vi "Dashboard Main Old.vi"() -> ()   [LabVIEW 2015]
uses:
  <vilib>/Utility/miscctls.llb/LVRowAndColumnTypeDef.ctl
  <vilib>/event_ctls.llb/eventvkey.ctl
  <vilib>/Rock Robotics/WPI/Dashboard/WPI_DashboardLogging Global.vi
  <vilib>/Rock Robotics/Network Tables/NT Write Boolean.vi
  <vilib>/Utility/config.llb/Write Key (String).vi
  <vilib>/Utility/config.llb/Write Key (I32).vi
  <vilib>/Utility/config.llb/NI_LVConfig.lvlib
panel:
  in  "TCP":refnum<k5>
  in  "Rec Mode":enum32{"Stop", "Record", "Playback"}(radio)
  in  "Vision":u16(ring)=2 items=["Camera Off", "USB Camera SW", "USB Camera HW", "IP Camera"]
  out "Camera IP":string
  out "Image Message":string="Timeout in Camera Communications"
  in  "Dashboard Tab":T1(tab)
  out "NT Connection":bool
  in  "Camera Settings":T2={"Frame Rate"=30, "Compression"=30, "Size"=1} {"Frame Rate" scale=1.0..30.0; "Size" items=["640x480", "320x240", "160x120"]}
  out "Gyro":dbl(knob) scale=0.0..360.0
  out "Mode":T3(ring)=enum."Auto Disabled"
  in  "DB Camera Config":bool
  out "fps":dbl format="%#.1g"
  out "Mbps":dbl format="%#.1g"
  out "Mbps LED":bool
  in  "DB/String 9":string
  in  "DB/String 8":string
  in  "DB/String 7":string
  in  "DB/String 6":string
  in  "DB/String 5":string
  in  "DB/String 4":string
  in  "DB/String 3":string
  in  "DB/String 2":string
  in  "DB/String 1":string
  in  "DB/String 0":string
  in  "DB/Slider 0":dbl(slide) scale=0.0..5.0
  in  "DB/Slider 1":dbl(slide) scale=0.0..5.0
  in  "DB/Slider 2":dbl(slide) scale=0.0..5.0
  in  "DB/Slider 3":dbl(slide) scale=0.0..5.0
  out "DB/LED 3":bool
  out "DB/LED 2":bool
  out "DB/LED 1":bool
  out "DB/LED 0":bool
  in  "DB/Button 3":bool
  in  "DB/Button 2":bool
  in  "DB/Button 1":bool
  in  "DB/Button 0":bool caption="New Name"
  in  "Auto Mode":u16(ring) items=["Do Nothing", "Drive to OW", "Drive through OW", "Shoot"]
  in  "Select Auto":string(combo)="Do Nothing"
  in  "Starting Position":u16(ring) items=["1", "2", "3", "4", "5", "Spy"]
  in  "Defense to Cross":u16(ring) items=["Low Bar", "Moat", "Ramparts", "Rock Wall", "Rough Terrain", "Cheval", "Portculis"]
  in  "Shooter Towards Defense":bool
  in  "Test Slider":dbl(slide) scale=0.0..100.0 scale format="%#_3g"
  in  "On/Off":bool caption="Solenoid"
  in  "Test Name":u16(ring) items=["Select the test to run..."]
  in  "Test Tree":string(tree)
  in  "Motor":cluster{"Value":dbl, "Enable":bool} {"Value" scale=-1.0..1.0 scale format="%#_3g"}
  out "Progress":T4 {"Test Progress" scale=0.0..100.0}
  in  "Rev/Fwd":cluster{"Forward":bool, "Reverse":bool}
  in  "Test Ring":u16(ring) items=["Monochrome", "Color"]
  out "Cmd Status":string
  in  "Execute Command":bool
  in  "Command Params":string[][](table)
  in  "Command Selection":i32(listbox)
  in  "CheckList":i32(listbox)
  out "Tree":string(tree)
  out "Camera Image":T5(plugin-control)
  out "Background":bool
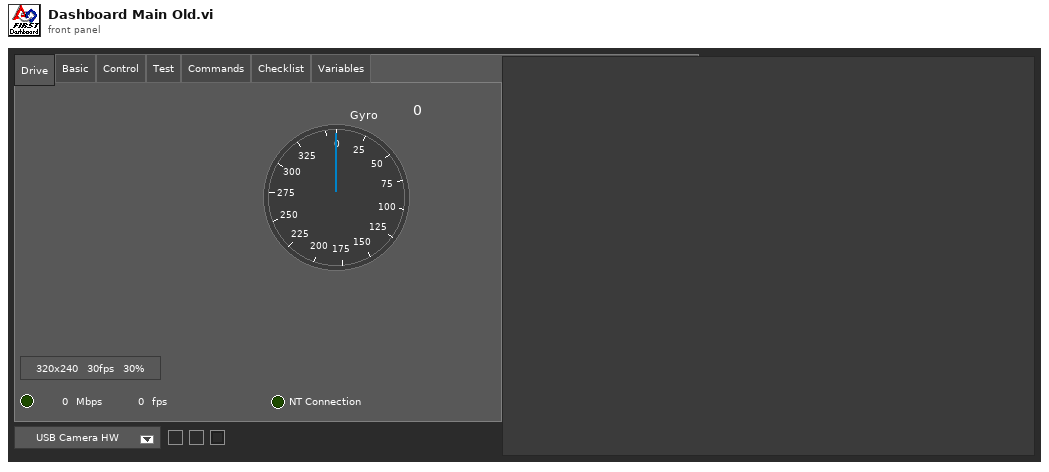
[diagram p1: front panel]
types:
  T1 = enum32{"Drive", "Basic", "Control", "Test", "Commands", "Checklist", "Variables"}
  T2 = cluster{"Frame Rate":i32, "Compression":i32, "Size":u16}
  T3 = enum8{"Tele-Op Disabled", "Tele-Op Enabled", "Auto Disabled", "Auto Enabled", "Test Disabled", "Test Enabled", "Disconnected", "No Code", "E-Stop"}
  T4 = cluster{"Test Progress":u8, "Test Progress Text":string}
  T5 = typedef "IMAQ Image.ctl" = refnum<image>
  T6 = cluster{"IDs":cluster{"RPC field ID":u16, "Unique ID":u16}, "String":string}
  T7 = enum32{"Drive", "Basic", "Custom", "Test", "Checklist", "Variables"}
  T8 = typedef "Image Type" = u32
  T9 = cluster{"Camera Image":refnum<vi>, "Dashboard Tab":refnum<vi>, "Background":refnum<vi>, "Vision":refnum<vi>, "Rec Mode":refnum<vi>, "Test Slider":refnum<vi>, "On/Off ":refnum<vi>, "Test Ring":refnum<vi>, "Rev/Fwd":refnum<vi>, "Test Name":refnum<vi>, "Motor":refnum<vi>, "Progress":refnum<vi>, "CheckList":refnum<vi>, "Tree":refnum<vi>, "Test Tree":refnum<vi>, "Command Params":refnum<vi>, "Command Selection":refnum<vi>, "Execute Command":refnum<vi>, "Cmd Status":refnum<vi>}
  T10 = cluster{"Error Strings":string, "Disable Counts":cluster{u16, u16}, "Rail Faults":cluster{u16, u16, u16}, "Robot IP":string, "DB Mode":u8, "Event Info":cluster{"Name":string, "Type":u8, "Number":u16, "Replay":u8}, "Camera Addr":string}
  T11 = cluster{"Storage":cluster{"Disk Free":u64, "RAM Block":u32, "RAM free":u32}, "CPU Utilization":cluster{"CPU % ISR":sgl, "CPU % Time Crit":sgl, "CPU % Timed Str":sgl, "CPU % High":sgl, "CPU % Above":sgl, "CPU % Normal":sgl, "CPU % Low":sgl}, "CAN":cluster{"% Bus Utilization":sgl, "Bus Off Cnt":u32, "TX_FIFO Full Cnt":u32, "Receive Error Cnt":u8, "Transmit Error Cnt":u8}, "HID":cluster{"HID Outputs":u32, "Rumble Low":u16, "Rumble High":u16}[]}
  T12 = cluster{"Status bits":cluster{"Test Mode":bool, "Autonomous":bool, "Enabled":bool, "Code Start":bool, "Brownout":bool, "Reserved 2":bool, "Reserved 3":bool, "E-Stop":bool}, "Code Trace":cluster{"Disabled":bool, "TeleOp":bool, "Auto":bool, "Test":bool}, "Controller Type":enum16{"unknown", "cRIO", "roboRio"}, "Code?":enum16{"unknown", "noCode", "code"}, "Battery V":dbl}
  T13 = cluster{"Control Bits":cluster{"TestMode":bool, "Autonomous":bool, "Enabled":bool, "FMS Present":bool, bool, bool, bool, "E-Stop":bool}, "Team Station ":u8, "Countdown":sgl, "Joystick Values":cluster{"Axes":dbl[], "Buttons":bool[], "POVs":i16[]}[]}
  T14 = typedef "NI_LVConfig.lvlib/Config Data RefNum.ctl" = refnum<k1>
  T15 = cluster{"Operation":enum16{"Update", "Clear"}, "Color Box":u32}[]
  T16 = typedef "eventvkey.ctl" = enum16{"ASCII", "Enter", "Return", "Shift", "Ctrl", "Alt", "Cmd", "Opt", "Caps", "NumLock", "Clear", "Break", "Up", "Down", "Left", "Right", "Insert", "Delete", "Home", "End", "PageUp", "PageDown", "Escape", "Help", "Pause", "ScrollLock", "F1", "F2", "F3", "F4", "F5", "F6", "F7", "F8", "F9", "F10", "F11", "F12", "F13", "F14", "F15", "F16", "F17", "F18", "F19", "F20", "F21", "F22", "F23", "F24", "Play", "VolumeUp", "VolumeDown", "Mute", "Two Byte Char"}
  T17 = cluster{"Image Size":bool, "Image Type":bool, "Pixel Value":bool, "ROI Information":bool, "Zoom Factor":bool}
  T18 = enum8{"Enabled", "Disabled", "Disabled and Grayed Out"}
  T19 = cluster{"Operation":enum16{"Update", "Clear"}, "Color Box":u32}
  T20 = typedef "LVRowAndColumnTypeDef.ctl" = cluster{"Row":i32, "Column":i32}
  T21 = cluster{"Shift":bool, "Ctrl":bool, "Alt":bool, "Cmd":bool, "Opt":bool}
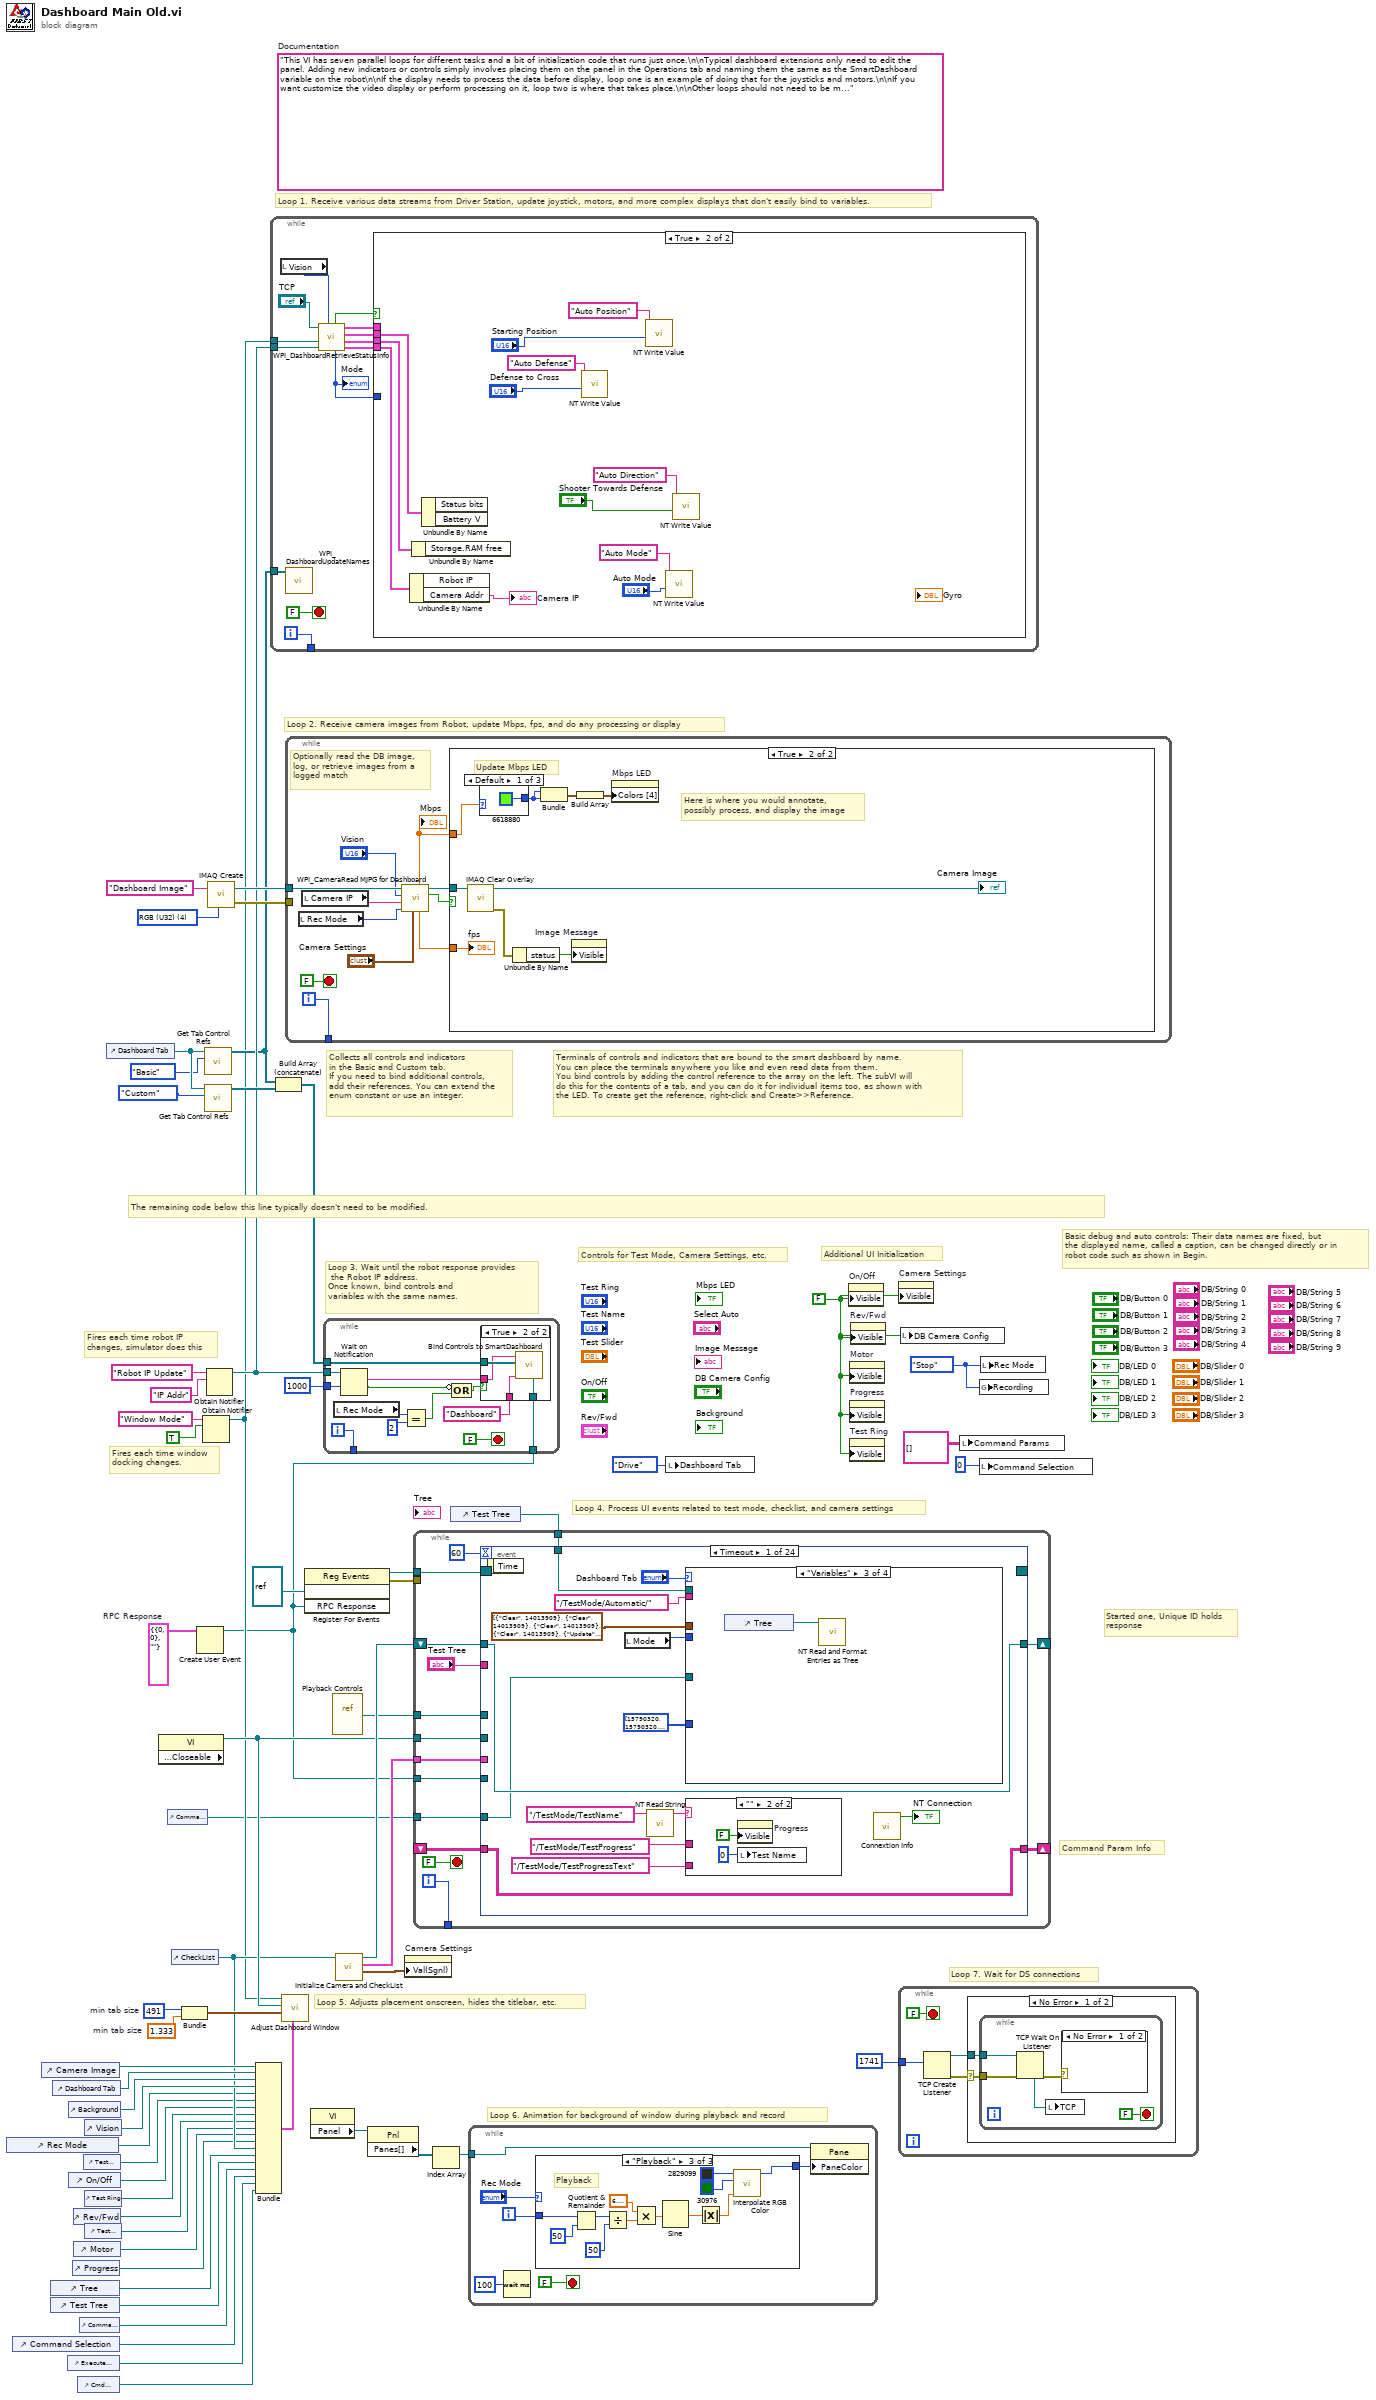
[diagram p0: block diagram]
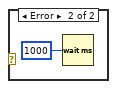
[diagram p2: hidden frame]
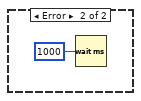
[diagram p3: hidden frame]
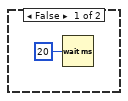
[diagram p4: hidden frame]
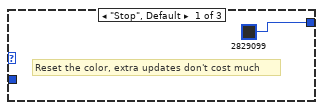
[diagram p5: hidden frame]
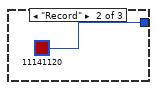
[diagram p6: hidden frame]
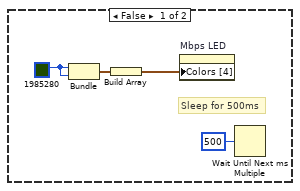
[diagram p8: hidden frame]
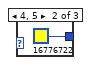
[diagram p9: hidden frame]
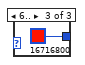
[diagram p10: hidden frame]
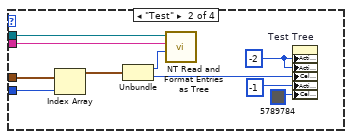
[diagram p12: hidden frame]
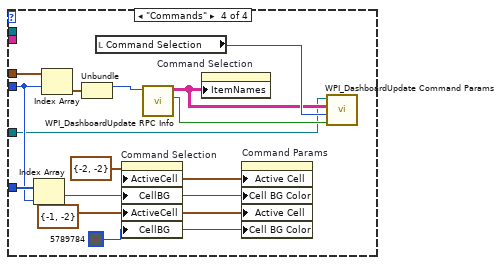
[diagram p13: hidden frame]
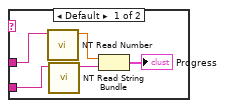
[diagram p14: hidden frame]
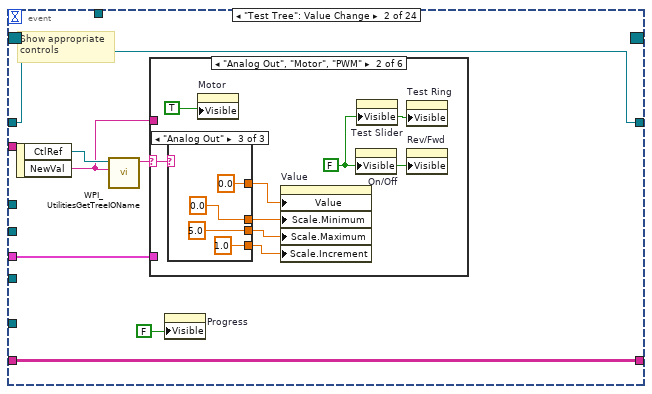
[diagram p15: hidden frame]
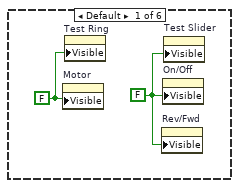
[diagram p16: hidden frame]
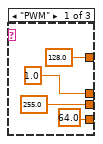
[diagram p17: hidden frame]
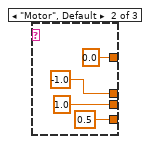
[diagram p18: hidden frame]
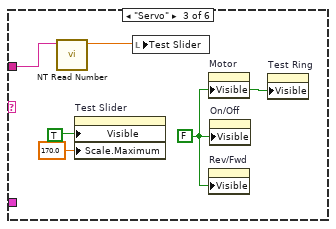
[diagram p19: hidden frame]
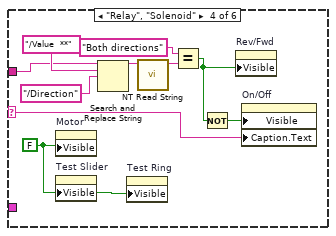
[diagram p20: hidden frame]
diagram:
  w8 = T6 {"IDs"={"RPC field ID"=0, "Unique ID"=0}, "String"=""}  # RPC Response
  w33 = 491  # min tab size
  w32 = 1.333  # min tab size
  w41 = enum32{"Stop", "Record", "Playback"}."Stop" ("Rec Mode")
  w15 = FALSE ("Visible")
  (unwired) "This VI has seven parallel loops for different tasks and a bit of initialization code that runs just once.\n\nTypical dashboard extensions only need to edit the panel. Adding new indicators or controls simply involves placing them on the panel in the Operations tab and naming them the same as the SmartDashboard variable on the robot\n\nIf the display needs to process the data before display, loop one is an example of doing that for the joysticks and motors.\n\nIf you want customize the video display or perform processing on it, loop two is where that takes place.\n\nOther loops should not need to be modified. They are pretty standard, and document the task they perform."  # Documentation
  w61 = T8 4 items=["Grayscale (U8)", "Grayscale (I16)", "Grayscale (SGL)", "Complex (CSG)", "RGB (U32)", "HSL (U32)", "RGB (U64)"] ("Image Type")
  # "Command Param Info"
  # "Started one, Unique ID holds\nresponse"
  # "Loop 7. Wait for DS connections"
  # "Basic debug and auto controls: Their data names are fixed, but\nthe displayed name, called a caption, can be changed directly or in\nrobot code such as shown in Begin."
  # "Controls for Test Mode, Camera Settings, etc."
  # "Additional UI Initialization"
  # "Loop 6. Animation for background of window during playback and record"
  # "Fires each time robot IP\nchanges, simulator does this"
  # "Fires each time window\ndocking changes."
  # "Collects all controls and indicators\nin the Basic and Custom tab.\nIf you need to bind additional controls,\nadd their references. You can extend the\nenum constant or use an integer."
  # "The remaining code below this line typically doesn't need to be modified."
  # "Loop 4. Process UI events related to test mode, checklist, and camera settings"
  # "Terminals of controls and indicators that are bound to the smart dashboard by name.\nYou can place the terminals anywhere you like and even read data from them.\nYou bind controls by adding the control reference to the array on the left. The subVI will\ndo this for the contents of a tab, and you can do it for individual items too, as shown with\nthe LED. To create get the reference, right-click and Create>>Reference."
  # "Loop 3. Wait until the robot response provides\n the Robot IP address.\nOnce known, bind controls and\nvariables with the same names."
  # "Loop 5. Adjusts placement onscreen, hides the titlebar, etc."
  # "Loop 1. Receive various data streams from Driver Station, update joystick, motors, and more complex displays that don't easily bind to variables."
  # "Loop 2. Receive camera images from Robot, update Mbps, fps, and do any processing or display"
  n1 = control-ref of="Rec Mode"() -> (w21:refnum<vi>)
  n2 = control-ref of="Command Selection"() -> (w7:refnum<vi>)
  n3 = control-ref of="Camera Image"() -> (w36:refnum<vi>)
  n4 = control-ref of="Tree"() -> (w25:refnum<vi>)
  n5 = control-ref of="Test Tree"() -> (w24:refnum<vi>)
  n6 = control-ref of="Dashboard Tab"() -> (w35:refnum<vi>)
  n7 = control-ref of="Execute Command"() -> (w9:refnum<vi>)
  n8 = control-ref of="Background"() -> (w30:refnum<vi>)
  n9 = control-ref of="On/Off"() -> (w19:refnum<vi>)
  n10 = control-ref of="Progress"() -> (w16:refnum<vi>)
  n11 = control-ref of="Rev/Fwd"() -> (w17:refnum<vi>)
  n12 = control-ref of="Motor"() -> (w22:refnum<vi>)
  n13 = control-ref of="Cmd Status"() -> (w3:refnum<vi>)
  n14 = control-ref of="Command Params"() -> (w10:refnum<vi>)
  n15 = control-ref of="Test Slider"() -> (w20:refnum<vi>)
  n16 = control-ref of="Vision"() -> (w34:refnum<vi>)
  n17 = control-ref of="Test Ring"() -> (w18:refnum<vi>)
  n18 = control-ref of="Test Name"() -> (w23:refnum<vi>)
  n19 = control-ref of="Dashboard Tab"() -> (w39:refnum<vi>)
  n20 = property class="VI" props=["Front Panel.Closeable"]() -> (reference out=w40:refnum<vi>)  [unwired: 2 in, 2 out]
  n21 = control-ref of="Command Params"() -> (w2:refnum<vi>)
  n22 = control-ref of="CheckList"() -> (w26:refnum<vi>)
  n23 = Bundle("min tab size"=w33, "min tab size"=w32) -> (w31:cluster{"min tab size":i32, "min tab size":dbl})  [unwired: 1 in]
  n24 = Create User Event(user event datatype=w8) -> (user event=w4:refnum<user-event>)  [unwired: 1 in, 1 out]
  n25 = Obtain Notifier(name (unnamed)="Window Mode", notification data type=TRUE) -> (notifier out=w12:refnum<notifier>)  [unwired: 2 in, 2 out]
  n26 = call <vilib>:"Get Tab Control Refs.vi"("Page Index"=T7."Basic" ("Dashboard Tab"), "TabControl in"=w39) -> ("ControlsOnPage"=w13:refnum<vi>[])  [unwired: 9 in]
  n27 = call <vilib>:"Get Tab Control Refs.vi"("Page Index"=T7."Custom" ("Dashboard Tab"), "TabControl in"=w39) -> ("ControlsOnPage"=w38:refnum<vi>[])  [unwired: 9 in]
  n28 = Obtain Notifier(name (unnamed)="Robot IP Update", notification data type="IP Addr" ("name (unnamed)")) -> (notifier out=w14:refnum<notifier>)  [unwired: 2 in, 2 out]
  n29 = call "IMAQ Create"("Image Name"="Dashboard Image", "Image Type"=w61) -> ("New Image"=w59:T5, "error out"=w58:errorcluster)  [unwired: 2 in, 1 out]
  n30 = Bundle("Camera Image"=w36, "Dashboard Tab"=w35, "Background"=w30, "Vision"=w34, "Rec Mode"=w21, "Test Slider"=w20, "On/Off"=w19, "Test Ring"=w18, "Rev/Fwd"=w17, "Test Name"=w23, "Motor"=w22, "Progress"=w16, "CheckList"=w26, "Tree"=w25, "Test Tree"=w24, "Command Params"=w10, "Command Selection"=w7, "Execute Command"=w9, "Cmd Status"=w3) -> (w27:T9)  [unwired: 1 in]
  n31 = while {
    tunnel: [w73] -> _
    tunnel: w14 -> [w67]
    tunnel: w13 -> [w66]
    tunnel: w12 -> [w62]
    i -> [w73]
    stop <- FALSE stop-if-true
    n32 = local read "Vision"() -> (w64:u16)
    n33 = call <vilib>:"WPI_DashboardUpdateNames.vi"("Controls on Tab"=w66) -> ()  [unwired: 11 in]
    n34 = call <vilib>:"WPI_DashboardRetrieveStatusInfo.vi"("Vision"=w64, "Binding Refnum"=w67, "Window Mode Notifier"=w62, "TCP Cnx"="TCP") -> ("Power and Errors"=w68:T10, "Robot Metrics"=w71:T11, "Status Info"=w72:T12, "Control Info"=w69:T13, "Robot Mode"=w65:T3, "Process?"=w70:bool)  [unwired: 2 in]
    "Mode" <- w65
    n35 = case shown="True" w70 {
      tunnel: w72 -> [_ w87]
      tunnel: w71 -> [_ w86]
      tunnel: w69 -> [_ _]
      tunnel: w68 -> [_ w85]
      tunnel: w65 -> [_ _]
      frame False {
        n36 = Wait (ms)(milliseconds to wait=u32 20) -> ()  [unwired: 1 out]
      }
      frame True {
        n37 = Unbundle By Name(w85) -> ("Camera Addr"=→"Camera IP":string)  [unwired: 1 out]
        n38 = Unbundle By Name(w86) -> ()  [unwired: 1 out]
        n39 = Unbundle By Name(w87) -> ()  [unwired: 2 out]
        n40 = call-poly <vilib>:"NT Write Value.vi"("Numeric"="Defense to Cross", "Name"="Auto Defense") -> ()  [unwired: 9 in, 1 out]
        n41 = call-poly <vilib>:"NT Write Value.vi"("Numeric"="Starting Position", "Name"="Auto Position") -> ()  [unwired: 9 in, 1 out]
        n42 = call-poly <vilib>:"NT Write Value.vi"("Numeric"="Auto Mode", "Name"="Auto Mode") -> ()  [unwired: 9 in, 1 out]
        n43 = call-poly <vilib>:"NT Write Value.vi"("Boolean"="Shooter Towards Defense", "Name"="Auto Direction") -> ()  [unwired: 9 in, 1 out]
      }
    }
  }
  n44 = Build Array (concatenate)(w13, w38) -> (w37:refnum<vi>[])
  n45 = call "Adjust Dashboard Window.vi"("Sizing Refnums"=w27, "Size Constraints"=w31, "VI"=w40, "WIn Mode"=w12) -> ()  [unwired: 8 in]
  n46 = while {
    tunnel: w59 -> [w96]
    tunnel: w58 -> [_]
    tunnel: [w97] -> _
    i -> [w97]
    stop <- FALSE stop-if-true
    # "Optionally read the DB image,\nlog, or retrieve images from a\nlogged match"
    n47 = local read "Rec Mode"() -> (w91:enum32{"Stop", "Record", "Playback"})
    n48 = local read "Camera IP"() -> (w89:string)
    n49 = call <vilib>:"WPI_CameraRead MJPG for Dashboard.vi"("Camera Settings"="Camera Settings", "Rec Mode"=w91, "Camera IP"=w89, "Camera Mode"="Vision", "Refnum in"=w96) -> ("Active"=w94:bool, "Refnum out"=w95:T5, "FPS"=w93:dbl, "Bandwidth (Mbps)"=w88:dbl)  [unwired: 3 in]
    "Mbps" <- w88
    n50 = case shown="True" w94 {
      tunnel: w95 -> [_ w106]
      tunnel: w88 -> [_ w105]
      tunnel: w93 -> [_ w104]
      frame False {
        w99 = u32 1985280 ("Color Box")
        # "Sleep for 500ms"
        n51 = Bundle("Color Box"=w99, "Color Box"=w99) -> (w101:cluster{"Color Box":u32, "Color Box":u32})  [unwired: 1 out]
        n52 = Build Array(w101) -> (w100:cluster{"Color Box":u32, "Color Box":u32}[])
        n53 = property on="Mbps LED" class="Bool (strict)"("Colors [4]"=w100) -> ()  [unwired: 2 in, 2 out]
        n54 = Wait Until Next ms Multiple(millisecond multiple=u32 500) -> ()  [unwired: 1 out]
      }
      frame True {
        # "Here is where you would annotate,\npossibly process, and display the image"
        # "Update Mbps LED"
        n55 = call "IMAQ Clear Overlay"("Image"=w106) -> ("error out"=w110:errorcluster, "Image Out"=→"Camera Image":T5)  [unwired: 2 in, 7 out]
        n56 = case shown="Default" w105 {
          tunnel: [u32 6618880 ("Color Box") u32 16776722 ("Color Box") u32 16716800 ("Color Box")] -> w107
          frame Default {
          }
          frame 4, 5 {
          }
          frame 6.. {
          }
        }
        n57 = Unbundle By Name(w110) -> ("status"=w111:bool)
        n58 = Bundle("Color Box"=w107, "Color Box"=w107) -> (w109:cluster{"Color Box":u32, "Color Box":u32})  [unwired: 1 out]
        n59 = property on="Image Message" class="Str"("Visible"=w111) -> ()  [unwired: 2 in, 2 out]
        n60 = Build Array(w109) -> (w108:cluster{"Color Box":u32, "Color Box":u32}[])
        n61 = property on="Mbps LED" class="Bool (strict)"("Colors [4]"=w108) -> ()  [unwired: 2 in, 2 out]
        "fps" <- w104
      }
    }
  }
  n62 = register-events(refnum<vi> refnum, w4) -> (reference out=w45:refnum<event-registration>, error out=w44:errorcluster)  [unwired: 2 in]
  n63 = property class="VI"() -> ("Panel"=w48:refnum<vi>)  [unwired: 2 in, 2 out]
  n64 = while {
    tunnel: w37 -> [w127]
    tunnel: w14 -> [w125]
    tunnel: [w123] -> _
    tunnel: u32 1000 ("milliseconds to wait") -> [w122]
    tunnel: w4 -> [w115]
    i -> [w123]
    stop <- FALSE stop-if-true
    n65 = local read "Rec Mode"() -> (w118:enum32{"Stop", "Record", "Playback"})
    n66 = Wait on Notification(notifier=w125, timeout in ms (-1)=w122) -> (notification=w124:string, timed out?=w120:bool)  [unwired: 2 in, 2 out]
    n67 = Equal?(x=w118, y=u16 2 ("Rec Mode")) -> (x = y?=w119:bool)
    n68 = Compound Arithmetic op=OR(invert w120, w119) -> (w121:bool)
    n69 = case shown="True" w121 {
      tunnel: w127 -> [_ w131]
      tunnel: w124 -> [_ w130]
      tunnel: "Dashboard" -> [_ w129]
      tunnel: w115 -> [_ w128]
      frame False {
      }
      frame True {
        n70 = call <vilib>:"Bind Controls to SmartDashboard.vi"("RPC ref"=w128, "Client Name"=w129, "Bound Control Refs"=w131, "Server IP Address"=w130) -> ()  [unwired: 8 in]
      }
    }
  }
  n71 = vi-ref "Playback Controls.vi"() -> (w46:refnum<vi>)
  n72 = call "Initialize Camera and CheckList.vi"("ListBox in"=w26) -> ("Cluster"=w52:cluster{"value":i32, "value":i32, "index":i32}, "Array"=w53:cluster{string[]}[], "File Refnum"=w51:T14)  [unwired: 8 in]
  n73 = property class="Pnl"(reference=w48) -> ("Panes[]"=w49:refnum<vi>[])  [unwired: 1 in, 2 out]
  n74 = property on="Camera Settings" class="Clust (strict)"("Val(Sgnl)"=w52) -> ()  [unwired: 2 in, 2 out]
  n75 = Index Array(array=w49) -> (element=w47:refnum<vi>)  [unwired: 1 in]
  n76 = control-ref of="Test Tree"() -> (w50:refnum<vi>)
  n77 = while {
    tunnel: w53 -> [w143]
    shift-right: [w142] -> _
    shift-left: w51 -> [w141]
    tunnel: [w140] -> _
    tunnel: w50 -> [w139]
    tunnel: w46 -> [w138]
    tunnel: w45 -> [w137]
    tunnel: w44 -> [_]
    tunnel: w40 -> [w136]
    tunnel: w4 -> [w135]
    tunnel: w2 -> [w134]
    shift-right: [w133] -> _
    shift-left: _ -> [w132]
    i -> [w140]
    stop <- FALSE stop-if-true
    n78 = event shown="[0] Timeout" {
      selector: w137 -> [_ _ _ _ _ _ _ _ _ _ _ _ _ _ _ _ _ _ _ _ _ _ _ _]
      dyn-events: [_ _ _ _ _ _ _ _ _ _ _ _ _ _ _ _ _ _ w452 _ _ _ _ _] -> _
      timeout: u32 60 ("milliseconds to wait") -> [_ _ _ _ _ _ _ _ _ _ _ _ _ _ _ _ _ _ _ _ _ _ _ _]
      tunnel: w139 -> [w156 _ _ _ _ _ _ _ _ _ _ _ _ _ _ _ _ _ _ _ _ _ _ _]
      tunnel: "Test Tree" -> [_ _ _ _ _ _ _ _ _ _ _ _ _ w415 w424 w427 w432 w441 _ _ _ _ _ _]
      tunnel: w143 -> [_ w194 _ _ _ _ _ _ _ _ _ w377 w408 _ _ _ _ _ _ _ _ _ _ _]
      tunnel: [w153 w193 w297 w303 w313 w317 w323 w335 w343 w349 w362 w376 w401 w414 w422 w426 w431 w440 w454 w470 w472 w480 w491 w496] -> w142
      tunnel: w141 -> [w153 w193 w297 w303 w313 w317 w323 w335 w343 w349 w362 w375 w401 w414 w422 w426 w431 w440 w454 w470 w472 w480 w491 w496]
      tunnel: w138 -> [_ _ _ _ _ _ _ _ _ _ _ _ _ _ _ _ _ _ w455 _ w475 _ _ _]
      tunnel: w136 -> [_ _ _ _ _ _ _ _ _ _ _ _ _ _ _ _ _ _ w450 _ _ _ _ _]
      tunnel: w135 -> [_ _ _ _ _ _ _ _ _ _ _ _ _ _ _ _ _ _ w446 _ _ _ _ _]
      tunnel: w134 -> [w148 _ _ _ _ _ w321 _ _ _ _ _ _ _ _ _ _ _ _ _ _ _ _ _]
      tunnel: [w147 w192 w296 w302 w312 w318 w319 w329 w340 w348 w361 w374 w400 w413 w421 w425 w430 w439 w445 w468 w471 w476 w484 w497] -> w133
      tunnel: w132 -> [w147 w192 w296 w302 w312 w318 w319 _ _ w348 w361 w374 w400 w413 w421 w425 w430 w439 w445 w468 w471 w476 w484 w497]
      event Timeout {
        n79 = event-data() -> ()  [unwired: 1 in, 1 out]
        n80 = local read "Mode"() -> (w150:T3)
        n81 = call <vilib>:"NT Read String.vi"("Name"="/TestMode/TestName") -> ("String"=w159:string)  [unwired: 9 in, 1 out]
        n82 = case shown="\"Variables\"" "Dashboard Tab" {
          tunnel: w156 -> [_ w170 _ _]
          tunnel: "/TestMode/Automatic/" ("Name Pattern") -> [_ w169 _ _]
          tunnel: T15 [{"Operation"=enum."Clear", "Color Box"=14013909}, {"Operation"=enum."Clear", "Color Box"=14013909}, {"Operation"=enum."Clear", "Color Box"=14013909}, {"Operation"=enum."Clear", "Color Box"=14013909}, {"Operation"=enum."Update", "Color Box"=14013909}, {"Operation"=enum."Update", "Color Box"=16777215}, {"Operation"=enum."Clear", "Color Box"=14013909}, {"Operation"=enum."Clear", "Color Box"=14013909}, {"Operation"=enum."Clear", "Color Box"=14013909}] -> [_ w162 _ w179]
          tunnel: w150 -> [_ w161 _ w178]
          tunnel: u32[] [15790320, 15790320, 15790320, 15790320, 16777215, 16777215, 15790320, 15790320, 15790320] -> [_ _ _ w184]
          tunnel: w148 -> [_ _ _ w172]
          frame "Control", Default {
          }
          frame "Test" {
            w168 = -2 ("Active Item:Row Number")
            n83 = Index Array(array=w162, index=w161) -> (element=w163:T19)
            n84 = Unbundle(w163) -> ("Operation"=w164:enum16{"Update", "Clear"}, "Color Box"=w165:u32)
            n85 = call <vilib>:"NT Read and Format Entries as Tree.vi"("Operation"=w164, "Name Pattern"=w169, "Tree Refnum"=w170) -> ()  [unwired: 7 in, 2 out]
            n86 = property on="Test Tree" class="Tree (strict)"("Active Item Row Number"=w168, "ActiveColNum"=w168, "CellBG"=w165, "Active Item Row Number"=-1 ("Active Item:Row Number"), "CellBG"=u32 5789784 ("Color Box")) -> ()  [unwired: 2 in, 2 out]
          }
          frame "Variables" {
            n87 = control-ref of="Tree"() -> (w171:refnum<vi>)
            n88 = call <vilib>:"NT Read and Format Entries as Tree.vi"("Tree Refnum"=w171) -> ()  [unwired: 9 in, 2 out]
          }
          frame "Commands" {
            w180 = u32 5789784 ("Color Box")
            w181 = T20 {"Row"=-1, "Column"=-2} ("Active Cell:Active Cell")
            w183 = T20 {"Row"=-2, "Column"=-2} ("Active Cell:Active Cell")
            n89 = Index Array(array=w184, index=w178) -> (element=w182:u32)
            n90 = Index Array(array=w179, index=w178) -> (element=w177:T19)
            n91 = Unbundle(w177) -> ("Operation"=w176:enum16{"Update", "Clear"})  [unwired: 1 out]
            n92 = local read "Command Selection"() -> (w175:i32)
            n93 = property on="Command Selection" class="MCListbox (strict)"("ActiveCell"=w183, "CellBG"=w182, "ActiveCell"=w181, "CellBG"=w180) -> ()  [unwired: 2 in, 2 out]
            n94 = call <vilib>:"WPI_DashboardUpdate RPC Info.vi"("Operation"=w176) -> ("update"=w174:bool, "commands"=w173:string[][])  [unwired: 9 in]
            n95 = property on="Command Selection" class="MCListbox (strict)"("ItemNames"=w173) -> ()  [unwired: 2 in, 2 out]
            n96 = property on="Command Params" class="Tbl (strict)"("Active Cell"=w183, "Cell BG Color"=w182, "Active Cell"=w181, "Cell BG Color"=w180) -> ()  [unwired: 2 in, 2 out]
            n97 = call <vilib>:"WPI_DashboardUpdate Command Params.vi"("Update"=w174, "NewVal"=w175, "Commands"=w173, "Param Tbl"=w172) -> ()  [unwired: 7 in, 1 out]
          }
        }
        n98 = case shown="\"\"" w159 {
          tunnel: "/TestMode/TestProgress" ("Name") -> [w186 _]
          tunnel: "/TestMode/TestProgressText" ("Name") -> [w185 _]
          frame Default {
            n99 = call <vilib>:"NT Read Number.vi"("Name"=w186) -> ("Numeric"=w187:dbl)  [unwired: 9 in, 1 out]
            n100 = call <vilib>:"NT Read String.vi"("Name"=w185) -> ("String"=w188:string)  [unwired: 9 in, 1 out]
            n101 = Bundle("Numeric"=w187, "String"=w188) -> (→"Progress":cluster{"Numeric":dbl, "String":string})  [unwired: 1 in]
          }
          frame "" {
            n102 = property on="Progress" class="Clust (strict)"("Visible"=FALSE) -> ()  [unwired: 2 in, 2 out]
            n103 = local write "Test Name"(u16 0) -> ()
          }
        }
        n104 = call <vilib>:"Connextion Info.vi"() -> ("Connected"=→"NT Connection":bool)  [unwired: 10 in, 1 out]
      }
      event "Test Tree": Value Change {
        # "Show appropriate\ncontrols"
        n105 = event-data() -> ("CtlRef"=w197:refnum<vi>, "NewVal"=w195:string)  [unwired: 1 in]
        n106 = call <vilib>:"WPI_UtilitiesGetTreeIOName.vi"("NewVal"=w195, "TreeControl in"=w197) -> ("I/O Name"=w198:string)  [unwired: 9 in]
        n107 = case shown="\"Analog Out\", \"Motor\", \"PWM\"" w198 {
          selector: w198 -> [_ w205 _ w227 w236 _]
          tunnel: w195 -> [_ _ w224 w226 _ w243]
          tunnel: w194 -> [_ _ _ _ _ w242]
          frame Default {
            w200 = FALSE ("Visible")
            w199 = FALSE ("Visible")
            n108 = property on="Motor" class="Clust (strict)"("Visible"=w199) -> ()  [unwired: 2 in, 2 out]
            n109 = property on="Test Ring" class="Ring (strict)"("Visible"=w199) -> ()  [unwired: 2 in, 2 out]
            n110 = property on="Rev/Fwd" class="Clust (strict)"("Visible"=w200) -> ()  [unwired: 2 in, 2 out]
            n111 = property on="On/Off" class="Bool (strict)"("Visible"=w200) -> ()  [unwired: 2 in, 2 out]
            n112 = property on="Test Slider" class="Slide (strict)"("Visible"=w200) -> ()  [unwired: 2 in, 2 out]
          }
          frame "Analog Out", "Motor", "PWM" {
            w206 = FALSE ("Visible")
            n113 = case shown="\"Analog Out\"" w205 {
              tunnel: [1.0 ("Value") -1.0 ("Value") 0.0 ("Value")] -> w204
              tunnel: [255.0 ("Value") 1.0 ("Value") 5.0 ("Value")] -> w203
              tunnel: [128.0 ("Value") 0.0 ("Value") 0.0 ("Value")] -> w202
              tunnel: [64.0 ("Value") 0.5 ("Value") 1.0 ("Value")] -> w201
              frame "PWM" {
              }
              frame "Motor", Default {
              }
              frame "Analog Out" {
              }
            }
            n114 = property on="Motor" class="Clust (strict)"("Visible"=TRUE) -> ()  [unwired: 2 in, 2 out]
            n115 = property on="Value" class="Slide (strict)"("Value"=w202, "Scale.Minimum"=w204, "Scale.Maximum"=w203, "Scale.Increment"=w201) -> ()  [unwired: 2 in, 2 out]
            n116 = property on="On/Off" class="Bool (strict)"("Visible"=w206) -> ()  [unwired: 2 in, 2 out]
            n117 = property on="Test Slider" class="Slide (strict)"("Visible"=w206) -> ()  [unwired: 2 in, 2 out]
            n118 = property on="Test Ring" class="Ring (strict)"("Visible"=w206) -> ()  [unwired: 2 in, 2 out]
            n119 = property on="Rev/Fwd" class="Clust (strict)"("Visible"=w206) -> ()  [unwired: 2 in, 2 out]
          }
          frame "Servo" {
            w222 = FALSE ("Visible")
            n120 = call <vilib>:"NT Read Number.vi"("Name"=w224) -> ("Numeric"=w223:dbl)  [unwired: 9 in, 1 out]
            n121 = property on="Test Slider" class="Slide (strict)"("Visible"=TRUE, "Scale.Maximum"=170.0 ("Scale.Range:Maximum")) -> ()  [unwired: 2 in, 2 out]
            n122 = local write "Test Slider"(w223) -> ()
            n123 = property on="Motor" class="Clust (strict)"("Visible"=w222) -> ()  [unwired: 2 in, 2 out]
            n124 = property on="Rev/Fwd" class="Clust (strict)"("Visible"=w222) -> ()  [unwired: 2 in, 2 out]
            n125 = property on="On/Off" class="Bool (strict)"("Visible"=w222) -> ()  [unwired: 2 in, 2 out]
            n126 = property on="Test Ring" class="Ring (strict)"("Visible"=w222) -> ()  [unwired: 2 in, 2 out]
          }
          frame "Relay", "Solenoid" {
            w225 = FALSE ("Visible")
            n127 = property on="Motor" class="Clust (strict)"("Visible"=w225) -> ()  [unwired: 2 in, 2 out]
            n128 = property on="Test Slider" class="Slide (strict)"("Visible"=w225) -> ()  [unwired: 2 in, 2 out]
            n129 = Search and Replace String(input string=w226, search string="/Value  **", replace string="/Direction") -> (result string=w232:string)  [unwired: 5 in, 3 out]
            n130 = property on="Test Ring" class="Ring (strict)"("Visible"=w225) -> ()  [unwired: 2 in, 2 out]
            n131 = call <vilib>:"NT Read String.vi"("Name"=w232) -> ("String"=w230:string)  [unwired: 9 in, 1 out]
            n132 = Equal?(x="Both directions", y=w230) -> (x = y?=w228:bool)
            n133 = Not(x=w228) -> (.not. x?=w229:bool)
            n134 = property on="Rev/Fwd" class="Clust (strict)"("Visible"=w228) -> ()  [unwired: 2 in, 2 out]
            n135 = property on="On/Off" class="Bool (strict)"("Visible"=w229, "Caption.Text"=w227) -> ()  [unwired: 2 in, 2 out]
          }
          frame "Compressor", "Digital Out" {
            w235 = FALSE ("Visible")
            # "Get direction and finish"
            n136 = property on="Motor" class="Clust (strict)"("Visible"=w235) -> ()  [unwired: 2 in, 2 out]
            n137 = property on="Test Slider" class="Slide (strict)"("Visible"=w235) -> ()  [unwired: 2 in, 2 out]
            n138 = property on="Test Ring" class="Ring (strict)"("Visible"=w235) -> ()  [unwired: 2 in, 2 out]
            n139 = property on="On/Off" class="Bool (strict)"("Visible"=TRUE, "Caption.Text"=w236) -> ()  [unwired: 2 in, 2 out]
            n140 = property on="Rev/Fwd" class="Clust (strict)"("Visible"=FALSE) -> ()  [unwired: 2 in, 2 out]
          }
          frame "Camera" {
            n141 = call <vilib>:"Get Last Path Segment.vi"("String in"=w243) -> ("String out"=w244:string)  [unwired: 10 in]
            n142 = property on="On/Off" class="Bool (strict)"("Visible"=FALSE) -> ()  [unwired: 2 in, 2 out]
            n143 = property on="Motor" class="Clust (strict)"("Visible"=FALSE) -> ()  [unwired: 2 in, 2 out]
            n144 = property on="Rev/Fwd" class="Clust (strict)"("Visible"=FALSE) -> ()  [unwired: 2 in, 2 out]
            n145 = case shown="\"White Balance  **\"" w244 {
              tunnel: w243 -> [w250 w259 w268 w277 w286 _ w292]
              tunnel: w242 -> [w248 w256 w265 w274 w283 _ _]
              frame "Size  **" {
                n146 = Index Array(array=w248) -> (element=w247:cluster{string[]})  [unwired: 1 in]
                n147 = call <vilib>:"NT Read String.vi"("Name"=w250) -> ("String"=w249:string)  [unwired: 9 in, 1 out]
                n148 = Unbundle(w247) -> (w245:string[])
                n149 = Match First String(2:w245, 3:w249) -> (0:w246:i32)  [unwired: 1 out]
                n150 = property on="Test Ring" class="Ring (strict)"("Value"=w246, "Strings []"=w245) -> ()  [unwired: 2 in, 2 out]
                n151 = property on="Test Ring" class="Ring (strict)"("Visible"=TRUE) -> ()  [unwired: 2 in, 2 out]
                n152 = property on="Test Slider" class="Slide (strict)"("Visible"=FALSE) -> ()  [unwired: 2 in, 2 out]
              }
              frame "White Balance  **" {
                n153 = Index Array(array=w256, index=1) -> (element=w257:cluster{string[]})
                n154 = call <vilib>:"NT Read String.vi"("Name"=w259) -> ("String"=w258:string)  [unwired: 9 in, 1 out]
                n155 = Unbundle(w257) -> (w254:string[])
                n156 = Match First String(2:w254, 3:w258) -> (0:w253:i32)  [unwired: 1 out]
                n157 = property on="Test Ring" class="Ring (strict)"("Value"=w253, "Strings []"=w254) -> ()  [unwired: 2 in, 2 out]
                n158 = property on="Test Ring" class="Ring (strict)"("Visible"=TRUE) -> ()  [unwired: 2 in, 2 out]
                n159 = property on="Test Slider" class="Slide (strict)"("Visible"=FALSE) -> ()  [unwired: 2 in, 2 out]
              }
              frame "Exposure  **" {
                n160 = Index Array(array=w265, index=2) -> (element=w266:cluster{string[]})
                n161 = call <vilib>:"NT Read String.vi"("Name"=w268) -> ("String"=w267:string)  [unwired: 9 in, 1 out]
                n162 = Unbundle(w266) -> (w262:string[])
                n163 = Match First String(2:w262, 3:w267) -> (0:w263:i32)  [unwired: 1 out]
                n164 = property on="Test Ring" class="Ring (strict)"("Value"=w263, "Strings []"=w262) -> ()  [unwired: 2 in, 2 out]
                n165 = property on="Test Ring" class="Ring (strict)"("Visible"=TRUE) -> ()  [unwired: 2 in, 2 out]
                n166 = property on="Test Slider" class="Slide (strict)"("Visible"=FALSE) -> ()  [unwired: 2 in, 2 out]
              }
              frame "Exposure Priority  **" {
                n167 = Index Array(array=w274, index=3) -> (element=w275:cluster{string[]})
                n168 = call <vilib>:"NT Read String.vi"("Name"=w277) -> ("String"=w276:string)  [unwired: 9 in, 1 out]
                n169 = Unbundle(w275) -> (w271:string[])
                n170 = Match First String(2:w271, 3:w276) -> (0:w272:i32)  [unwired: 1 out]
                n171 = property on="Test Ring" class="Ring (strict)"("Value"=w272, "Strings []"=w271) -> ()  [unwired: 2 in, 2 out]
                n172 = property on="Test Ring" class="Ring (strict)"("Visible"=TRUE) -> ()  [unwired: 2 in, 2 out]
                n173 = property on="Test Slider" class="Slide (strict)"("Visible"=FALSE) -> ()  [unwired: 2 in, 2 out]
              }
              frame "Color Enable  **" {
                n174 = Index Array(array=w283, index=4) -> (element=w284:cluster{string[]})
                n175 = call <vilib>:"NT Read String.vi"("Name"=w286) -> ("String"=w285:string)  [unwired: 9 in, 1 out]
                n176 = Unbundle(w284) -> (w280:string[])
                n177 = Match First String(2:w280, 3:w285) -> (0:w281:i32)  [unwired: 1 out]
                n178 = property on="Test Ring" class="Ring (strict)"("Value"=w281, "Strings []"=w280) -> ()  [unwired: 2 in, 2 out]
                n179 = property on="Test Ring" class="Ring (strict)"("Visible"=TRUE) -> ()  [unwired: 2 in, 2 out]
                n180 = property on="Test Slider" class="Slide (strict)"("Visible"=FALSE) -> ()  [unwired: 2 in, 2 out]
              }
              frame Default {
                n181 = property on="Test Ring" class="Ring (strict)"("Visible"=FALSE) -> ()  [unwired: 2 in, 2 out]
                n182 = property on="Test Slider" class="Slide (strict)"("Visible"=FALSE) -> ()  [unwired: 2 in, 2 out]
              }
              frame "Brightness  **", "Color Level  **", "Compression  **", "FPS  **", "Sharpness  **" {
                n183 = call <vilib>:"NT Read Number.vi"("Name"=w292) -> ("Numeric"=w291:dbl)  [unwired: 9 in, 1 out]
                n184 = local write "Test Slider"(w291) -> ()
                n185 = property on="Test Slider" class="Slide (strict)"("Visible"=TRUE, "Scale.Maximum"=100.0 ("Scale.Range:Maximum")) -> ()  [unwired: 2 in, 2 out]
                n186 = property on="Test Ring" class="Ring (strict)"("Visible"=FALSE) -> ()  [unwired: 2 in, 2 out]
              }
            }
          }
        }
        n187 = property on="Progress" class="Clust (strict)"("Visible"=FALSE) -> ()  [unwired: 2 in, 2 out]
      }
      event "Test Name": Mouse Enter {
        # "Populate the ring with the list of tests"
        n188 = event-data() -> ()  [unwired: 1 in, 1 out]
        n189 = call <vilib>:"NT Read String Array.vi"("Name"="/TestMode/TestList") -> ("String Array"=w301:string[])  [unwired: 9 in, 1 out]
        n190 = Build Array (concatenate)("Select the test to run...", w301) -> (w300:string[])
        n191 = property on="Test Name" class="Ring (strict)"("Strings []"=w300) -> ()  [unwired: 2 in, 2 out]
      }
      event "Test Name": Value Change {
        w304 = FALSE ("Visible")
        # "Tell the robot the test name to run"
        n192 = event-data() -> ("NewVal"=w308:u16)  [unwired: 1 in]
        n193 = property on="Test Name" class="Ring (strict)"() -> ("Strings []"=w309:string[])  [unwired: 2 in, 2 out]
        n194 = local write "Progress"(T4 {"Test Progress"=0, "Test Progress Text"=""} ("Progress")) -> ()
        n195 = Index Array(array=w309, index=w308) -> (element=w307:string)
        n196 = call <vilib>:"NT Write String.vi"("String"=w307, "Name"="/TestMode/TestName") -> ()  [unwired: 9 in, 1 out]
        n197 = property on="Progress" class="Clust (strict)"("Visible"=TRUE) -> ()  [unwired: 2 in, 2 out]
        n198 = property on="Motor" class="Clust (strict)"("Visible"=w304) -> ()  [unwired: 2 in, 2 out]
        n199 = property on="Test Slider" class="Slide (strict)"("Visible"=w304) -> ()  [unwired: 2 in, 2 out]
        n200 = property on="On/Off" class="Bool (strict)"("Visible"=w304) -> ()  [unwired: 2 in, 2 out]
        n201 = property on="Rev/Fwd" class="Clust (strict)"("Visible"=w304) -> ()  [unwired: 2 in, 2 out]
        n202 = property on="Test Ring" class="Ring (strict)"("Visible"=w304) -> ()  [unwired: 2 in, 2 out]
      }
      event "Select Auto": Mouse Enter {
        # "Populate the combo box with the list of autonomous options"
        n203 = event-data() -> ()  [unwired: 1 in, 1 out]
        n204 = call <vilib>:"NT Read String Array.vi"("Name"="Auto List") -> ("String Array"=w311:string[])  [unwired: 9 in, 1 out]
        n205 = property on="Select Auto" class="CmbBox"("Strings[]"=w311) -> ()  [unwired: 2 in, 2 out]
      }
      event "Select Auto": Value Change {
        # "User modified the Auto Selection. Write to NT variable so robot knows."
        n206 = event-data() -> ("NewVal"=w315:string)  [unwired: 1 in]
        n207 = call <vilib>:"NT Write String.vi"("String"=w315, "Name"="Auto Selector") -> ()  [unwired: 9 in, 1 out]
      }
      event "Command Selection": Value Change {
        # "Get the params and show in table"
        n208 = event-data() -> ("NewVal"=w322:i32)  [unwired: 1 in]
        n209 = property on="Command Selection" class="MCListbox (strict)"() -> ("ItemNames"=w320:string[][])  [unwired: 2 in, 2 out]
        n210 = call <vilib>:"WPI_DashboardUpdate Command Params.vi"("NewVal"=w322, "Commands"=w320, "Param Tbl"=w321) -> ()  [unwired: 8 in, 1 out]
      }
      event "Execute Command": Value Change {
        # "Started one, Unique ID holds\nresponse"
        n211 = event-data() -> ()  [unwired: 1 in, 1 out]
        n212 = property on="Command Selection" class="MCListbox (strict)"() -> ("ItemNames"=w334:string[][])  [unwired: 2 in, 2 out]
        n213 = Index Array(array=w334, index (row)="Command Selection", index (col)=0) -> (element=w332:string)
        n214 = call <vilib>:"Invoke Commands.vi"("Command Params"="Command Params", "Function Name"=w332) -> ("Params"=w328:u8, "Started"=w327:bool)  [unwired: 7 in, 1 out]
        n215 = Array Subset(array="Command Params", length (row)=w328) -> (w329:string[][])  [unwired: 3 in]
        n216 = Select(t="Executing" ("Cmd Status"), s=w327, f="" ("Cmd Status")) -> (s? t:f=→"Cmd Status":string)
      }
      event "Command Selection": Double Click {
        n217 = event-data() -> ("Row"=w344:i32)  [unwired: 1 in]
        n218 = property on="Command Selection" class="MCListbox (strict)"() -> ("ItemNames"=w347:string[][])  [unwired: 2 in, 2 out]
        n219 = local read "Command Params"() -> (w342:string[][])
        n220 = Index Array(array=w347, index (row)=w344, index (col)=0) -> (element=w345:string)
        n221 = call <vilib>:"Invoke Commands.vi"("Command Params"=w342, "Function Name"=w345) -> ("Params"=w341:u8, "Started"=w336:bool)  [unwired: 7 in, 1 out]
        n222 = Array Subset(array=w342, length (row)=w341) -> (w340:string[][])  [unwired: 3 in]
        n223 = Select(t="Executing" ("Cmd Status"), s=w336, f="" ("Cmd Status")) -> (s? t:f=w337:string)
        n224 = local write "Cmd Status"(w337) -> ()
      }
      event "CheckList": Double Click {
        # "Shift clears all"
        # "Update symbols on the listbox"
        n225 = event-data() -> ("PlatMods.Shift"=w350:bool, "Row"=w352:i32)  [unwired: 1 in]
        n226 = case shown="True" w350 {
          tunnel: w352 -> [w356 _]
          tunnel: 1 -> [w355 _]
          frame False {
            n227 = property on="CheckList" class="LstBox (strict)"() -> ("Item Symbols"=w354:i32[])  [unwired: 2 in, 2 out]
            n228 = Replace Array Subset(array=w354, new element=w355, index=w356) -> (w353:i32[])
            n229 = property on="CheckList" class="LstBox (strict)"("Item Symbols"=w353) -> ()  [unwired: 2 in, 2 out]
          }
          frame True {
            w357 = 0 ("Top Row")
            n230 = property on="CheckList" class="LstBox (strict)"() -> ("Number of Rows"=w359:u32)  [unwired: 2 in, 2 out]
            n231 = Initialize Array(0, w359) -> (w358:i32[])
            n232 = property on="CheckList" class="LstBox (strict)"("Top Row"=w357, "Value"=w357, "Item Symbols"=w358) -> ()  [unwired: 2 in, 2 out]
          }
        }
      }
      event "CheckList": Key Down {
        # "Update symbols on the listbox\nLeft and right keys check and uncheck"
        n233 = event-data() -> ("VKey"=w364:T16)  [unwired: 1 in]
        n234 = case shown="\"Left\", \"Right\"" w364 {
          selector: w364 -> [w369 _]
          tunnel: eventvkey."Left" ("VKey") -> [w367 _]
          frame "Left", "Right" {
            n235 = Equal?(x=w367, y=w369) -> (x = y?=w368:bool)
            n236 = Select(t=0, s=w368, f=1) -> (s? t:f=w370:i32)
            n237 = property on="CheckList" class="LstBox (strict)"() -> ("Item Symbols"=w373:i32[])  [unwired: 2 in, 2 out]
            n238 = Replace Array Subset(array=w373, new element=w370, index="CheckList") -> (w372:i32[])
            n239 = property on="CheckList" class="LstBox (strict)"("Item Symbols"=w372) -> ()  [unwired: 2 in, 2 out]
          }
          frame Default {
          }
        }
      }
      event "DB Camera Config": Value Change {
        # "Show or hide the cluster of controls, store in ini file"
        n240 = event-data() -> ("NewVal"=w378:bool)  [unwired: 1 in]
        n241 = case shown="False" w378 {
          tunnel: w377 -> [w387 _]
          tunnel: [w380 w398] -> w376
          tunnel: w375 -> [w379 w398]
          frame False {
            w394 = "Camera"
            w397 = FALSE ("Visible")
            n242 = local read "Camera Settings"() -> (w386:T2)
            n243 = Index Array(array=w387) -> (element=w390:cluster{string[]})  [unwired: 1 in]
            n244 = Unbundle(w386) -> ("Frame Rate"=w385:i32, "Compression"=w384:i32, "Size"=w388:u16)
            n245 = Unbundle(w390) -> (w389:string[])
            n246 = Index Array(array=w389, index=w388) -> (element=w383:string)
            n247 = call-poly <vilib>:"Write Key.vi"("section"=w394, "value"=w383, "key"="Size", "refnum"=w379) -> ("refnum out"=w396:T14)  [unwired: 2 in, 5 out]
            n248 = call-poly <vilib>:"Write Key.vi"("section"=w394, "value"=w385, "key"="FrameRate", "refnum"=w396) -> ("refnum out"=w395:T14)  [unwired: 1 in, 6 out]
            n249 = property on="Camera Settings" class="Clust (strict)"("Visible"=w397) -> ()  [unwired: 2 in, 2 out]
            n250 = local write "DB Camera Config"(w397) -> ()
            n251 = call-poly <vilib>:"Write Key.vi"("section"=w394, "value"=w384, "key"="Compression", "refnum"=w395) -> ("refnum out"=w381:T14)  [unwired: 1 in, 6 out]
            n252 = call <vilib>:"Close Config Data.vi"("refnum"=w381) -> ("file path"=w382:path)  [unwired: 2 in, 8 out]
            n253 = call <vilib>:"Open Config Data.vi"("configuration file path"=w382) -> ("refnum"=w380:T14)  [unwired: 8 in, 2 out]
          }
          frame True {
            n254 = property on="Camera Settings" class="Clust (strict)"("Visible"=TRUE) -> ()  [unwired: 2 in, 2 out]
          }
        }
      }
      event "Camera Settings": Value Change {
        # "Update summary string when any elements of DB camera change"
        n255 = event-data() -> ("NewVal"=w412:T2)  [unwired: 1 in]
        n256 = Index Array(array=w408) -> (element=w407:cluster{string[]})  [unwired: 1 in]
        n257 = Unbundle(w412) -> ("Frame Rate"=w403:i32, "Compression"=w402:i32, "Size"=w405:u16)
        n258 = Unbundle(w407) -> (w406:string[])
        n259 = Index Array(array=w406, index=w405) -> (element=w404:string)
        n260 = Format Into String(format string="%s   %dfps   %d%%", w404, w403, w402) -> (resulting string=w409:string)  [unwired: 2 in, 1 out]
        n261 = Build Array(w409) -> (w410:string[])
        n262 = property on="DB Camera Config" class="Bool (strict)"("Strings [4]"=w410) -> ()  [unwired: 2 in, 2 out]
      }
      event "Motor.Enable": Value Change {
        # "When the test mode otor enable helper is set, update that\ntree row item's value"
        n263 = event-data() -> ("NewVal"=w419:bool)  [unwired: 1 in]
        n264 = Unbundle("Motor") -> ("Value"=w418:dbl)  [unwired: 1 out]
        n265 = Select(t=w418, s=w419, f=0.0) -> (s? t:f=w416:dbl)
        n266 = call <vilib>:"NT Write Number.vi"("Numeric"=w416, "Name"=w415) -> ()  [unwired: 9 in, 1 out]
      }
      event "Test Slider": Value Change {
        # "When the test mode slider helper is set, update that\ntree row item's value"
        n267 = event-data() -> ("NewVal"=w423:dbl)  [unwired: 1 in]
        n268 = call <vilib>:"NT Write Number.vi"("Numeric"=w423, "Name"=w424) -> ()  [unwired: 9 in, 1 out]
      }
      event "On/Off": Value Change {
        # "When the test mode on/off helper value is set, update that\ntree row item's value"
        n269 = event-data() -> ("NewVal"=w429:bool)  [unwired: 1 in]
        n270 = Boolean To (0,1)(Boolean=w429) -> (0, 1=w428:i16)
        n271 = call <vilib>:"NT Write Number.vi"("Numeric"=w428, "Name"=w427) -> ()  [unwired: 9 in, 1 out]
      }
      event "Rev/Fwd": Value Change {
        # "When the test mode helper value for relays is set, update that\ntree row item's value"
        n272 = event-data() -> ("NewVal.Forward"=w438:bool, "NewVal.Reverse"=w437:bool)  [unwired: 1 in]
        n273 = Boolean To (0,1)(Boolean=w438) -> (0, 1=w434:i16)
        n274 = Boolean To (0,1)(Boolean=w437) -> (0, 1=w436:i16)
        n275 = Negate(x=w436) -> (-x=w435:i16)
        n276 = Add(x=w434, y=w435) -> (x+y=w433:i16)
        n277 = call <vilib>:"NT Write Number.vi"("Numeric"=w433, "Name"=w432) -> ()  [unwired: 9 in, 1 out]
      }
      event "Test Ring": Value Change {
        # "When a test mode helper value is selected from the ring,\nset the tree item's variable to the string value"
        n278 = event-data() -> ("NewVal"=w443:u16)  [unwired: 1 in]
        n279 = property on="Test Ring" class="Ring (strict)"() -> ("Strings []"=w444:string[])  [unwired: 2 in, 2 out]
        n280 = Index Array(array=w444, index=w443) -> (element=w442:string)
        n281 = call <vilib>:"NT Write String.vi"("String"=w442, "Name"=w441) -> ()  [unwired: 9 in, 1 out]
      }
      event "Rec Mode": Value Change {
        # "Update globals for recording mode and path to read log from.\nClear when logging and let NetworkTables set path for vision to\nuse."
        n282 = event-data() -> ("NewVal"=w456:enum32{"Stop", "Record", "Playback"})  [unwired: 1 in]
        n283 = global write "WPI_DashboardLogging Global.vi" "Logging Filename"(path "") -> ()
        n284 = global write "WPI_DashboardLogging Global.vi" "Recording"(w456) -> ()
        n285 = case shown="\"Playback\"" w456 {
          tunnel: w455 -> [_ w458 w467]
          tunnel: [_ _ w466] -> w452
          tunnel: [_ _ w465] -> _
          tunnel: w450 -> [_ _ w463]
          tunnel: cluster{i32, i32} {-250, 170} -> [_ _ w462]
          tunnel: [_ _ T17 {"Image Size"=TRUE, "Image Type"=TRUE, "Pixel Value"=TRUE, "ROI Information"=TRUE, "Zoom Factor"=FALSE} ("Image Information Shown:All Elements")] -> w448
          tunnel: [_ _ TRUE ("Zoom Factor")] -> w447
          tunnel: w446 -> [_ _ w459]
          frame Default {
          }
          frame "Stop", "Record" {
            # "Place Window too"
            n286 = invoke class="VI" method="FP.Close"(reference=w458) -> (reference out=w457:refnum<vi>)  [unwired: 2 in, 2 out]
            n287 = invoke class="VI" method="Abort VI"(reference=w457) -> ()  [unwired: 2 in, 3 out]
          }
          frame "Playback" {
            n288 = call "Open Playback Panel.vi"("Offset"=w462, "DB VI Ref"=w463, "Playback in"=w467) -> ("Playback out"=w464:refnum<vi>)  [unwired: 8 in]
            n289 = register-events(w464, w459) -> (reference out=w466:refnum<event-registration>, error out=w465:errorcluster)  [unwired: 2 in]
          }
        }
        n290 = property on="Camera Image" class="ImageControl"("Image Information Shown"=w448, "Image Information Visible"=w447) -> ()  [unwired: 2 in, 2 out]
        n291 = call <vilib>:"WPI_DashboardNT Log FieldName Cache.vi"("Operation"=enum16{"Lookup/Add", "Index", "Clear"}."Clear") -> ()  [unwired: 8 in, 3 out]
      }
      event Panel Close {
        w469 = enum32{"Stop", "Record", "Playback"}."Stop" ("Rec Mode")
        # "Playback window has been closed, abort"
        n292 = event-data() -> ()  [unwired: 1 in, 4 out]
        n293 = local write "Rec Mode"(w469) -> ()
        n294 = global write "WPI_DashboardLogging Global.vi" "Recording"(w469) -> ()
      }
      event Panel Close {
        # "Abort playback window and ourself"
        n295 = event-data() -> ()  [unwired: 1 in, 4 out]
        n296 = invoke class="VI" method="FP.Close"(reference=w475) -> (reference out=w474:refnum<vi>)  [unwired: 2 in, 2 out]
        n297 = invoke class="VI" method="Abort VI"(reference=w474) -> (error out=w473:errorcluster)  [unwired: 2 in, 2 out]
        n298 = invoke class="VI" method="Abort VI"(error in=w473) -> ()  [unwired: 2 in, 3 out]
      }
      event User Event {
        n299 = event-data() -> ("IDs"=w483:cluster{"RPC field ID":u16, "Unique ID":u16}, "String"=w482:string)  [unwired: 1 in]
        n300 = Bundle("IDs"=w483, "String"=w482) -> (w481:T6)  [unwired: 1 in]
        n301 = call <vilib>:"Retrieve RPC Response.vi"("RPC Response"=w481) -> ("Output"=w478:string[][])  [unwired: 10 in]
        n302 = Build Array (concatenate)(w476, w478) -> (w477:string[][])
        n303 = local write "Command Params"(w477) -> ()
        n304 = local write "Cmd Status"("" ("Cmd Status")) -> ()
      }
      event "Vision": Value Change {
        # "Enable/Disable Compression slider.\nHW USB is hard-coded into the camera"
        n305 = event-data() -> ("NewVal"=w490:u16)  [unwired: 1 in]
        n306 = Equal?(x=w490, y=u32 2 ("milliseconds to wait")) -> (x = y?=w488:bool)
        n307 = Select(t=T18."Disabled and Grayed Out" ("Disabled"), s=w488, f=T18."Enabled" ("Disabled")) -> (s? t:f=w485:T18)
        n308 = property on="Compression" class="Slide (strict)"("DisabledEnum"=w485) -> ()  [unwired: 2 in, 2 out]
      }
      event "Tree": Double Click {
        n309 = event-data() -> ("PlatMods"=w495:T21, "Tag"=w494:string)  [unwired: 1 in]
        n310 = Unbundle(w495) -> ("Shift"=w493:bool)  [unwired: 4 out]
        n311 = Not(x=w493) -> (.not. x?=w492:bool)
        n312 = call <vilib>:"NT Update Persistence.vi"("Persistence"=w492, "Name"=w494) -> ()  [unwired: 9 in, 1 out]
      }
    }
  }
  n313 = while {
    tunnel: w47 -> [w499]
    i -> [w502]
    stop <- FALSE stop-if-true
    n314 = Wait (ms)(milliseconds to wait=u32 100) -> ()  [unwired: 1 out]
    n315 = case shown="\"Playback\"" "Rec Mode" {
      tunnel: w502 -> [_ _ w517]
      tunnel: [u32 2829099 ("Base Color") u32 11141120 ("Target Color") w506] -> w498
      frame "Stop", Default {
        # "Reset the color, extra updates don't cost much"
      }
      frame "Record" {
      }
      frame "Playback" {
        # "Playback"
        n316 = Quotient & Remainder(x=w517, y=u32 50 ("milliseconds to wait")) -> (x-y*floor(x/y)=w513:u32)  [unwired: 1 out]
        n317 = Divide(x=w513, y=u32 50 ("milliseconds to wait")) -> (x/y=w510:dbl)
        n318 = Multiply(x=6.283185307179586, y=w510) -> (x*y=w515:dbl)
        n319 = Sine(x=w515) -> (sin(x)=w514:dbl)
        n320 = Absolute Value(x=w514) -> (abs(x)=w507:dbl)
        n321 = call "Interpolate RGB Color.vi"("Proportion"=w507, "Target Color"=u32 30976, "Base Color"=u32 2829099) -> ("Result Color"=w506:u32)  [unwired: 8 in]
      }
    }
    n322 = property class="Pane"(reference=w499, "PaneColor"=w498) -> ()  [unwired: 1 in, 2 out]
  }
  n323 = local write "Dashboard Tab"(T1."Drive" ("Dashboard Tab")) -> ()
  n324 = property on="On/Off" class="Bool (strict)"("Visible"=w15) -> ()  [unwired: 2 in, 2 out]
  n325 = property on="Motor" class="Clust (strict)"("Visible"=w15) -> ()  [unwired: 2 in, 2 out]
  n326 = property on="Progress" class="Clust (strict)"("Visible"=w15) -> ()  [unwired: 2 in, 2 out]
  n327 = property on="Test Ring" class="Ring (strict)"("Visible"=w15) -> ()  [unwired: 2 in, 2 out]
  n328 = property on="Rev/Fwd" class="Clust (strict)"("Visible"=w15) -> ()  [unwired: 2 in, 2 out]
  n329 = property on="Camera Settings" class="Clust (strict)"("Visible"=w15) -> ()  [unwired: 2 in, 2 out]
  n330 = while {
    tunnel: u16 1741 ("timeout ms (25000)") -> [w519]
    stop <- FALSE stop-if-true
    n331 = TCP Create Listener(10:w519) -> (0:w518:errorcluster, 3:w520:refnum<k5>)  [unwired: 4 in, 1 out]
    n332 = case shown="No Error" w518 {
      selector: w518 -> [w522 _]
      tunnel: w520 -> [w523 _]
      frame No Error {
        n333 = while {
          tunnel: w523 -> [w526]
          tunnel: w522 -> [w525]
          stop <- FALSE stop-if-true
          n334 = TCP Wait On Listener(8:w525, 11:w526) -> (0:w527:errorcluster, 4:w528:refnum<k5>)  [unwired: 2 in, 3 out]
          n335 = local write "TCP"(w528) -> ()
          n336 = case shown="No Error" w527 {
            frame No Error {
            }
            frame Error {
              n337 = Wait (ms)(milliseconds to wait=u32 1000) -> ()  [unwired: 1 out]
            }
          }
        }
      }
      frame Error {
        n338 = Wait (ms)(milliseconds to wait=u32 1000) -> ()  [unwired: 1 out]
      }
    }
  }
  n339 = local write "DB Camera Config"(w15) -> ()
  n340 = local write "Command Params"(string[][] [] ("Command Params")) -> ()
  n341 = global write "WPI_DashboardLogging Global.vi" "Recording"(w41) -> ()
  n342 = local write "Command Selection"(u16 0 ("milliseconds to wait")) -> ()
  n343 = local write "Rec Mode"(w41) -> ()
